vi "Group Data Type.vi"(8 "error in (no error)":errorcluster, 11 "Group in":refnum<class "Group.lvclass">) -> (0 "error out":errorcluster, 2 "Group Data Type":T1, 3 "Group out":refnum<class "Group.lvclass">)   [LabVIEW 2020, in "Vecto.lvlib" / "Group.lvclass"]
uses:
  Group.lvclass
  Group Data Type.ctl
  Vecto.lvlib
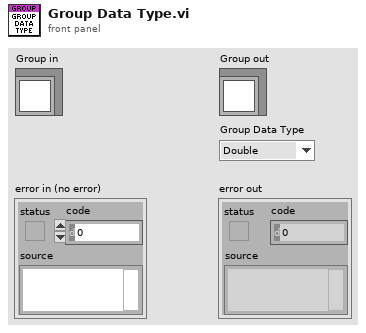
[diagram p1: front panel]
types:
  T1 = typedef "Vecto.lvlib/Group Data Type.ctl" = enum16{"Double", "String"}
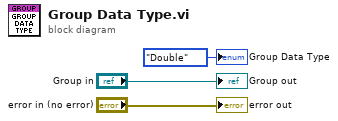
[diagram p0: block diagram]
diagram:
  "error out" <- "error in (no error)"
  "Group out" <- "Group in"
  "Group Data Type" <- Group_Data_Type."Double" ("Group Data Type")
